vi "定时启动对话框.vi"() -> (2 "设置值":dbl, 3 "确定输出":bool)   [LabVIEW 2016, in "斯坦道总磷总氮.lvlib"]
panel:
  in  "停止":bool
  in  "确定":bool
  in  "数值":dbl
  # "请输入定时启动间隔"
  # "min"
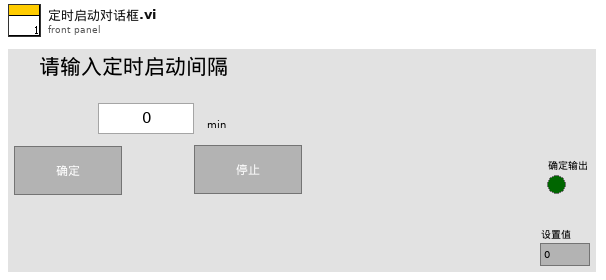
[diagram p1: front panel]
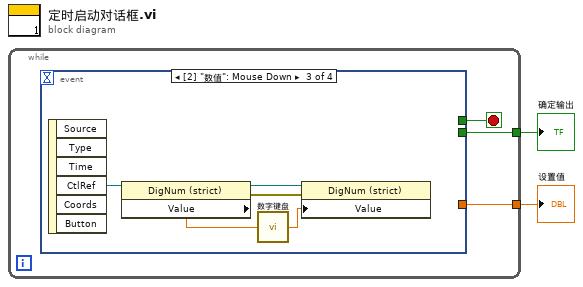
[diagram p0: block diagram]
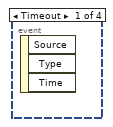
[diagram p2: hidden frame]
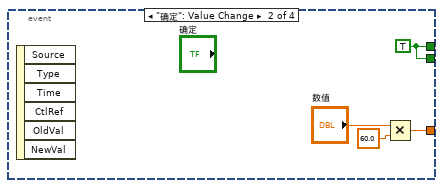
[diagram p3: hidden frame]
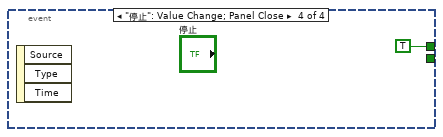
[diagram p4: hidden frame]
diagram:
  n1 = while {
    tunnel: [w5] -> w1
    tunnel: [w3] -> w2
    stop <- w4 stop-if-true
    n2 = event shown="[2] \"数值\": Mouse Down" {
      selector: _ -> [_ _ _ _]
      dyn-events: _ -> [_ _ _ _]
      timeout: _ -> [_ _ _ _]
      tunnel: [_ w7 _ _] -> w5
      tunnel: [_ w6 _ TRUE ("确定")] -> w4
      tunnel: [_ w6 _ _] -> w3
      event Timeout {
        n3 = event-data() -> ()  [unwired: 1 in, 3 out]
      }
      event "确定": Value Change {
        w6 = TRUE ("确定")
        n4 = event-data() -> ()  [unwired: 1 in, 6 out]
        n5 = Multiply(x="数值", y=60.0) -> (x*y=w7:dbl)
      }
      event "数值": Mouse Down {
        n6 = event-data() -> ("CtlRef"=w14:refnum<vi>)  [unwired: 1 in, 5 out]
        n7 = property class="DigNum (strict)"(reference=w14) -> (reference out=w13:refnum<vi>, error out=w12:errorcluster, "Value"=w11:dbl)  [unwired: 1 in]
        n8 = call "数字键盘.vi"("OldNumber"=w11) -> ("NewNumber"=w10:dbl)
        n9 = property class="DigNum (strict)"(reference=w13, error in=w12, "Value"=w10) -> ()  [unwired: 2 out]
      }
      event "停止": Value Change; Panel Close {
        n10 = event-data() -> ()  [unwired: 1 in, 3 out]
      }
    }
  }
  "确定输出" <- w2
  "设置值" <- w1
